vi "Read Ultramat 6EF 2 channel.vi"() -> ()   [LabVIEW 2021]
uses:
  Data Model/ELAN Data Model/Type Definitions/Value full.ctl
  Data Unit/ELAN PC Data Unit/Elan units.ctl
  Data Unit/ELAN PC Data Unit/Elan measured variable.ctl
  Data Unit/ELAN PC Data Unit/Elan channel state.ctl
  Transmission Data Unit/ELAN/ELAN Data Unit.lvclass
  Network Protocol/ELAN Master/ELAN Master.lvclass
  Transmission Data Unit/ELAN/ELAN Data Unit.lvclass/ELAN Data Unit.ctl
  Network Protocol/ELAN Master/ELAN Master.lvclass/ELAN Master.ctl
  Data Unit/ELAN PC Data Unit/ELAN PDU.lvclass
  Data Model/ELAN Data Model/ELAN Data Model.lvclass
panel:
  out "connect 2":bool
  out "connect":bool
  out "Value 2":T1 {"Value"."Value" format="%#_6f"}
  out "Value":T1 {"Value"."Value" format="%#_6f"}
  in  "visa resource name":refnum<visa-resource-name>="COM19"
  in  "Component address 2":u8=32 format="%x"
  in  "stop":bool
  in  "Component address":u8=16 format="%x"
  out "error out":errorcluster
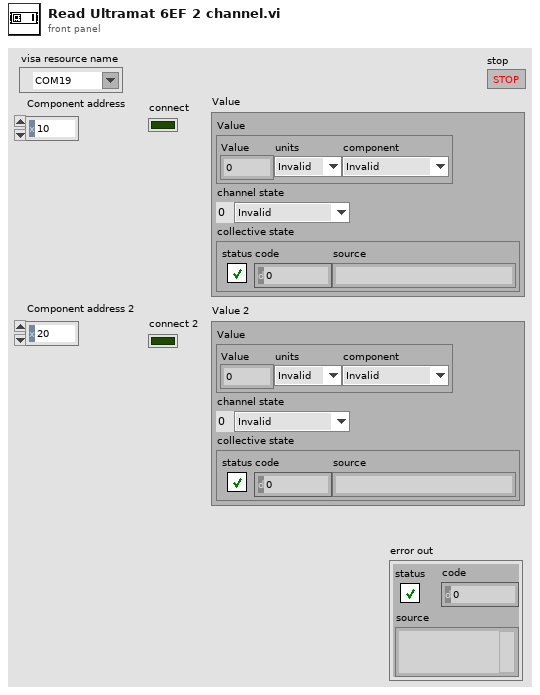
[diagram p1: front panel]
types:
  T1 = typedef "ELAN Data Model.lvclass/Value full.ctl" = cluster{"Value":cluster{"Value":sgl, "units":T2, "component":T3}, "channel state":T4, "collective state":errorcluster}
  T2 = typedef "ELAN PDU.lvclass/Elan units.ctl" = enum16{"Invalid", "no dimension", "ppm", "ppb", "vpm", "ppm C1", "ppm C3", "ppm C6", "mg C/m3", "mg/m3", "%", "% vol", "% of measuring range", "% saturation", "%/°C", "%/K", "% weight", "mV/pH", "mV/mbar", "nA/mbar", "S/m", "S/cm", "mS/m", "mS/cm", "ìS/m", "ìS/cm", "S", "min", "H", "Pa", "MA", "uV", "MV", "V", "mbar", "hPa", "Ml/min", "kOhm", "MOhm", "S1", "°C", "Hz", "pH", "ug/l", "mg/l", "l/min", "uA", "mg/dm3", "kPa", "kOhm*cm", "MOhm*cm", "°", "1/min", "1/m", "g/m3", "g/l", "% Vol C"}
  T3 = typedef "ELAN PDU.lvclass/Elan measured variable.ctl" = enum16{"Invalid", "no component", "CO", "CO2", "CH4 (Methan)", "C6H14 (Hexan)", "SO2", "NO", "NO2", "CHClF2 (R22)", "C3H8 (Propan)", "C4H10 (Butan)", "O2", "C5H12 (Pentan)", "CnHm (THC)", "P (process pressure)", "pH", "T (temperature)", "C2H4 (Ethen)", "C2H2 (Ethin)", "C3H6 (Propen)", "C4H6", "C4H8", "C2H6", "NH3 (Ammoniak)", "N2O", "C6H6 (Benzol)", "SF6", "CH3OH (Methanol)", "C2H5OH (Ethanol)", "CH2Cl2", "C2H4Cl2", "CH3Cl", "C2H4O", "H2O (water vapor)", "G/l (conductivity)", "C", "S", "N", "CF4", "COCl2 (phosgene)", "CHF3 (R23)", "C2F6 (R116)", "------ (self defined component)", "C2H3Cl", "H2 (Hydrogen)", "Ar", "He", "Cl2", "N2"}
  T4 = typedef "ELAN PDU.lvclass/Elan channel state.ctl" = enum16{"Invalid", "Warm-up", "Pause", "Standby", "Measure", "Zero calibration", "Adjust component slope", "Not yet defined1", "Adjust curve dip", "Adjust linearization sensitivity", "Adjust temperature compensation", "Adjust pressure compensation", "Adjust linearization zero", "Not yet defined2", "Autocal", "Adjust phase", "Zero calibration of O2 sensor", "Synchronous zero calibration", "Purging for synchronous zero calibration", "Adjust analog output", "Adjust analog input", "Autocal check"}
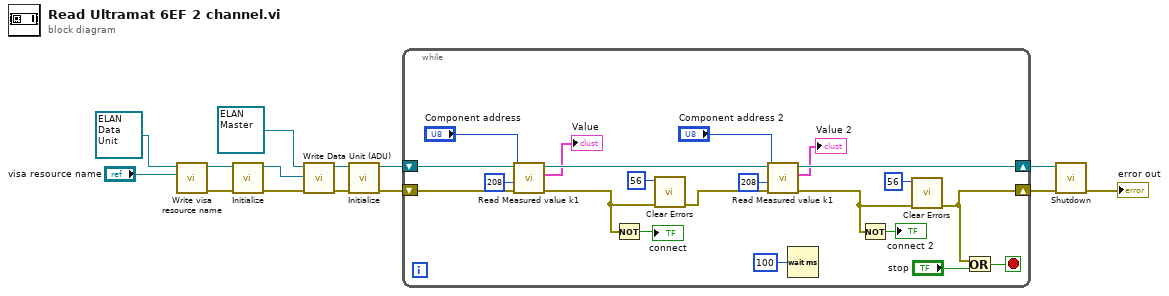
[diagram p0: block diagram]
diagram:
  n1 = call "Write visa resource name.vi"("visa resource name"="visa resource name", "ELAN Data Unit in"=refnum<class "ELAN Data Unit.lvclass"> refnum ("ASCII Data Unit")) -> ("error out"=w5:errorcluster, "ELAN Data Unit out"=w6:refnum<class "ELAN Data Unit.lvclass">)  [unwired: 8 in]
  n2 = call "Initialize.vi"("error in"=w5, "ELAN data unit (ADU) in"=w6) -> ("error out"=w13:errorcluster, "ELAN data unit (ADU) out"=w12:refnum<class "ELAN Data Unit.lvclass">)  [unwired: 8 in]
  n3 = call "Write Data Unit (ADU).vi"("error in (no error)"=w13, "ASCII Data Unit"=w12, "ELAN Master in"=refnum<class "ELAN Master.lvclass"> refnum) -> ("error out"=w10:errorcluster, "ELAN Master out"=w9:refnum<class "ELAN Master.lvclass">)  [unwired: 7 in]
  n4 = call-dynamic "Initialize.vi"("error in"=w10, "ELAN Master in"=w9) -> ("error out"=w8:errorcluster, "ELAN Master out"=w7:refnum<class "ELAN Master.lvclass">)  [unwired: 8 in]
  n5 = while {
    shift-right: [w21] -> w1
    shift-left: w8 -> [w35]
    shift-right: [w26] -> w2
    shift-left: w7 -> [w34]
    stop <- w22 stop-if-true
    n6 = call "Read Measured value k1.vi"("error in (no error)"=w35, "Control system address"=u8 208, "Component address"="Component address", "ELAN master in"=w34) -> ("error out"=w18:errorcluster, "Value"=→"Value":T1, "ELAN master out"=w27:refnum<class "ELAN Master.lvclass">)  [unwired: 4 in, 1 out]
    n7 = Not(x=w18) -> (.not. x?=→"connect":bool)
    n8 = call <vilib>:"Clear Errors.vi"("error in (no error)"=w18, "specific error code to clear (0: all)"=56) -> ("error out"=w25:errorcluster)  [unwired: 4 in, 1 out]
    n9 = call "Read Measured value k1.vi"("error in (no error)"=w25, "Control system address"=u8 208, "Component address"="Component address 2", "ELAN master in"=w27) -> ("error out"=w15:errorcluster, "Value"=→"Value 2":T1, "ELAN master out"=w26:refnum<class "ELAN Master.lvclass">)  [unwired: 4 in, 1 out]
    n10 = Wait (ms)(milliseconds to wait=u32 100 ("millisecond multiple")) -> ()  [unwired: 1 out]
    n11 = Not(x=w15) -> (.not. x?=→"connect 2":bool)
    n12 = call <vilib>:"Clear Errors.vi"("error in (no error)"=w15, "specific error code to clear (0: all)"=56) -> ("error out"=w21:errorcluster)  [unwired: 4 in, 1 out]
    n13 = Or(x=w21, y="stop") -> (x .or. y?=w22:bool)
  }
  n14 = call-dynamic "Shutdown.vi"("error in"=w1, "ELAN Master in"=w2) -> ("error out"=→"error out":errorcluster)  [unwired: 9 in]
